vi "DEV Check If File Already In Database.vi"() -> ()   [LabVIEW 2018, in "Database.lvlib"]
uses:
  Database.lvlib
panel:
  out "Already in Database?":bool
  in  "Path":path
  out "Error Out":errorcluster
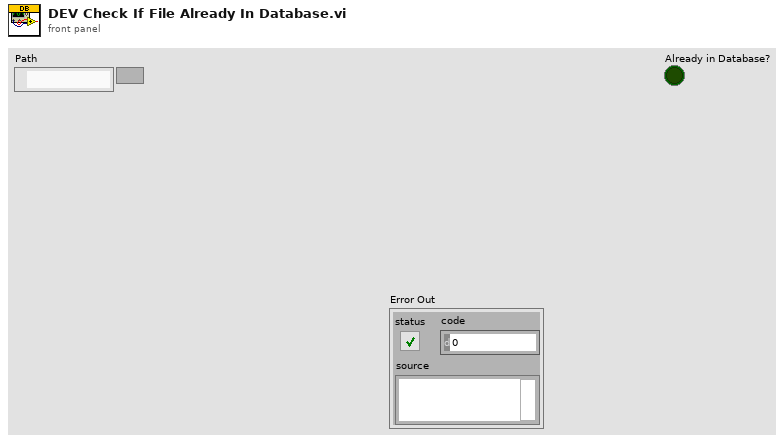
[diagram p1: front panel]
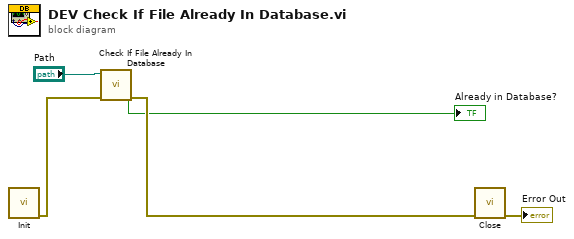
[diagram p0: block diagram]
diagram:
  n1 = call "Init.vi"() -> ("Error Out"=w5:errorcluster)  [unwired: 11 in]
  n2 = call "Check If File Already In Database.vi"("error in (no error)"=w5, "Path"="Path") -> ("error out"=w4:errorcluster, "Already in Database?"=→"Already in Database?":bool)  [unwired: 8 in]
  n3 = call "Close.vi"("Error In"=w4) -> ("Error Out"=→"Error Out":errorcluster)  [unwired: 10 in]
